vi "GraphsUpdateMai.vi"(0 "raw graph ref":refnum<vi>, 1 "File Paths":T3={"Local Save Path"=path "\\\\smbhome.uscs.susx.ac.uk\\cv222/Desktop/data", "Newton Save Path"=path "Z:/#Projects/Entanglement/data", "File Name"="test", "LocalSave"=TRUE}, 3 "Compiler Settings":T2={"Python Path"=path "", "Main File"="mainscript.py", "Meta File"="metascript.txt", "Aux File"="auxscript.py"}, 5 "mean graph ref":refnum<vi>, 7 "proc graph ref":refnum<vi>, 11 "error in (no error)":errorcluster, 12 "XControllerSettings":T1(xcontrol)) -> (15 "error out":errorcluster)   [LabVIEW 2017]
uses:
  controls/FilePaths.ctl
  PulseCompiler/CompilerSettings.ctl
  controls/xControllerSettings/XControllerSettings.xctl
  controls/GlobalExp.vi
  Global.lvlib
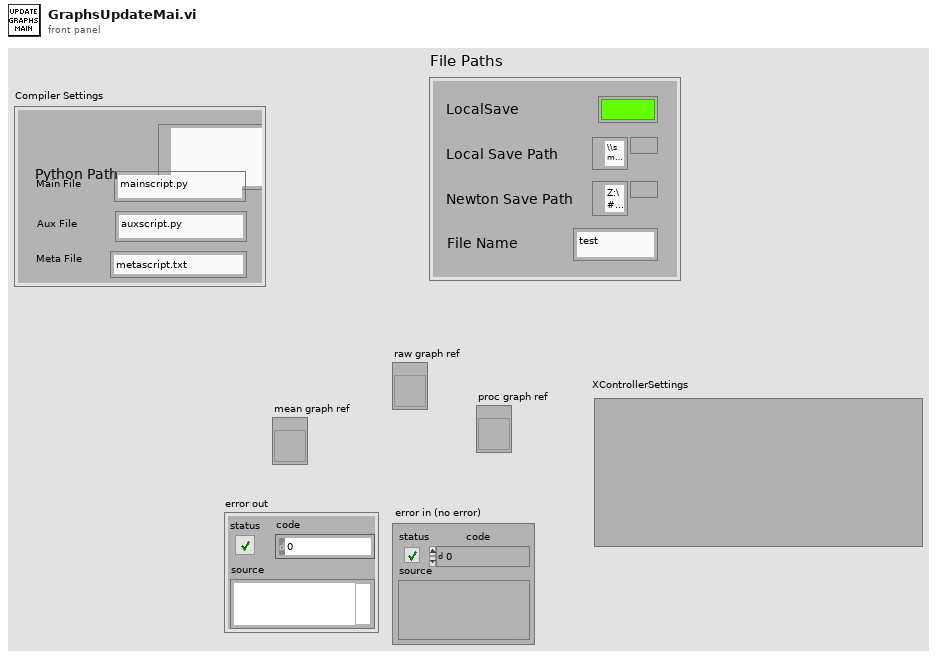
[diagram p1: front panel]
types:
  T1 = cluster{"Aux Sequence":bool, "Camera":bool, "Recrystallize":bool, "Raw graph":bool, "Mean graph":bool, "Calculate probs":bool, "Find fit":bool, "Dummy":bool}
  T2 = typedef "CompilerSettings.ctl" = cluster{"Python Path":path, "Main File":string, "Meta File":string, "Aux File":string}
  T3 = typedef "FilePaths.ctl" = cluster{"Local Save Path":path, "Newton Save Path":path, "File Name":string, "LocalSave":bool}
  T4 = typedef "MasterExpControl.ctl" = cluster{"Main Steps":dbl, "Main Runs":dbl, "ExpStatus":enum16{"Innit", "Stop", "Idle", "MainRunning", "AuxRunning"}, "Main Current Step":dbl, "ExpNum":dbl, "NewData":bool, "date":string, "command":string, "Stop":bool, "Pause":bool, "Mathematica":string, "Main/Meta":bool, "UpdateMath":bool, "Camera":bool, "MetaExpOver":bool}
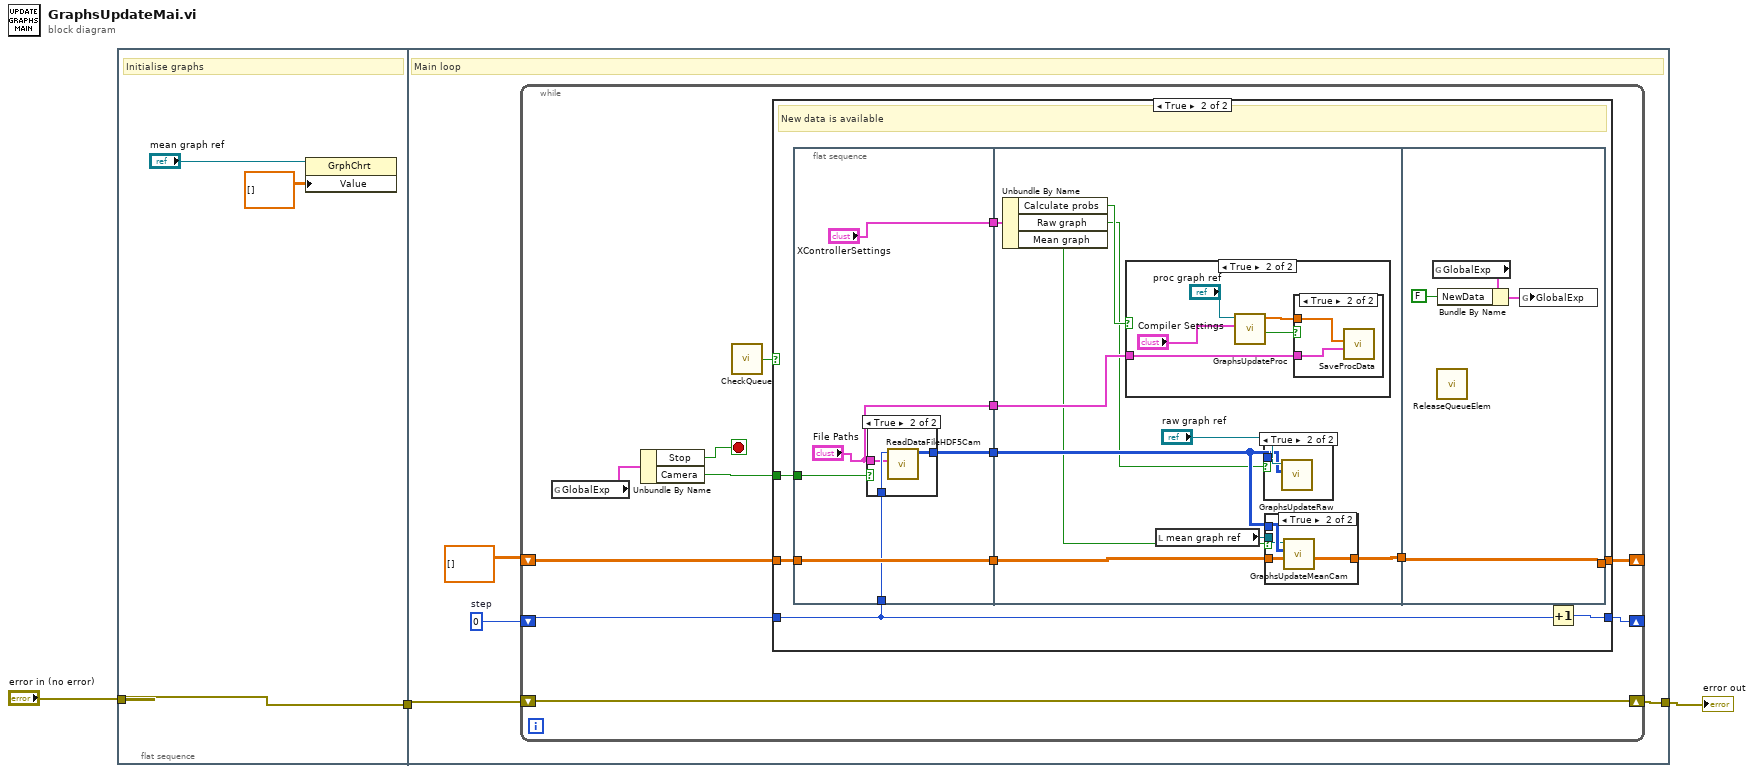
[diagram p0: block diagram]
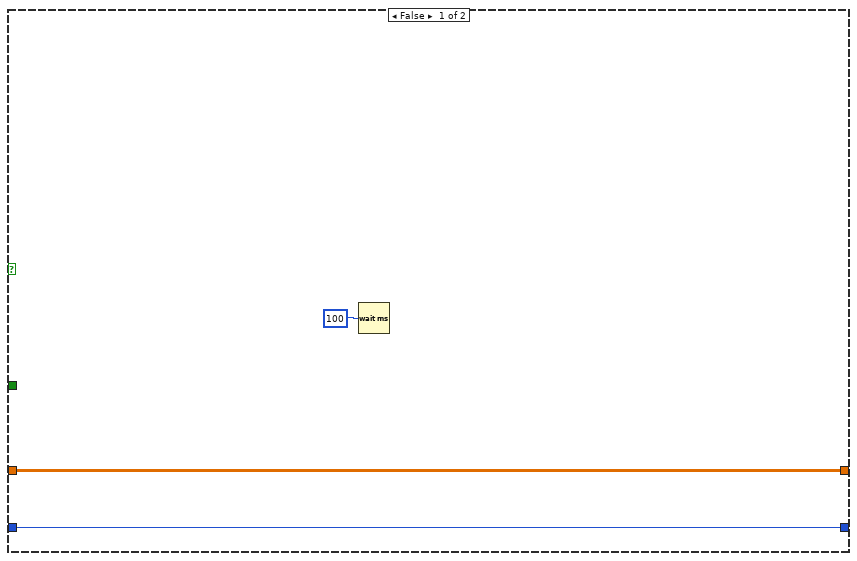
[diagram p2: hidden frame]
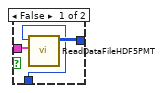
[diagram p3: hidden frame]
diagram:
  n1 = flat-sequence {
    tunnel: "error in (no error)" -> [w6]
    tunnel: [w6] -> w1
    tunnel: [w9] -> w2
    tunnel: w1 -> [w10]
    frame #0 {
      # "Initialise graphs"
      n2 = property class="GrphChrt"(reference="mean graph ref", "Value"=dbl[][] []) -> ()  [unwired: 1 in, 2 out]
    }
    frame #1 {
      w8 = 0  # step
      # "Main loop"
      n3 = while {
        shift-right: [w19] -> w9
        shift-left: w10 -> [w19]
        shift-right: [w13] -> _
        shift-left: w8 -> [w14]
        shift-right: [w11] -> _
        shift-left: dbl[][] [] -> [w12]
        stop <- w16 stop-if-true
        n4 = global read "GlobalExp.vi" "GlobalExp"() -> (w18:T4)
        n5 = Unbundle By Name(w18) -> ("Stop"=w16:bool, "Camera"=w17:bool)
        n6 = call "CheckQueue.vi"() -> ("x > 0?"=w15:bool)
        n7 = case shown="True" w15 {
          tunnel: w17 -> [_ w24]
          tunnel: w14 -> [w21 w29]
          tunnel: [w21 w32] -> w13
          tunnel: w12 -> [w20 w31]
          tunnel: [w20 w25] -> w11
          frame False {
            n8 = Wait (ms)(milliseconds to wait=u32 100) -> ()  [unwired: 1 out]
          }
          frame True {
            # "New data is available"
            n9 = flat-sequence {
              tunnel: w31 -> [w38]
              tunnel: [w38] -> w30
              tunnel: w29 -> [w37]
              tunnel: [w36] -> w28
              tunnel: ["File Paths"] -> w27
              tunnel: w24 -> [w34]
              tunnel: ["XControllerSettings"] -> w23
              tunnel: w30 -> [w54]
              tunnel: w28 -> [w51]
              tunnel: w27 -> [w52]
              tunnel: [w49] -> w26
              tunnel: w23 -> [w47]
              tunnel: w26 -> [w69]
              tunnel: [w69] -> w25
              frame #0 {
                n10 = case shown="True" w34 {
                  tunnel: w37 -> [w39 w44]
                  tunnel: [w41 w43] -> w36
                  tunnel: "File Paths" -> [w40 w42]
                  frame False {
                    n11 = call "ReadDataFileHDF5PMT.vi"("File Paths"=w40, "step"=w39) -> ("last step data"=w41:i32[][])  [unwired: 8 in, 1 out]
                  }
                  frame True {
                    n12 = call "ReadDataFileHDF5Cam.vi"("File Paths"=w42, "step"=w44) -> ("last step data"=w43:i32[][])  [unwired: 8 in, 1 out]
                  }
                }
              }
              frame #1 {
                n13 = Unbundle By Name(w47) -> ("Calculate probs"=w48:bool, "Raw graph"=w46:bool, "Mean graph"=w45:bool)
                n14 = case shown="True" w48 {
                  tunnel: w52 -> [_ w55]
                  frame False {
                  }
                  frame True {
                    n15 = call "GraphsUpdateProc.vi"("Compiler Settings"="Compiler Settings", "Prob graph ref in"="proc graph ref") -> ("SaveToCSV?"=w58:bool, "value"=w59:dbl[])  [unwired: 8 in]
                    n16 = case shown="True" w58 {
                      tunnel: w59 -> [_ w61]
                      tunnel: w55 -> [_ w60]
                      frame False {
                      }
                      frame True {
                        n17 = call "SaveProcData.vi"("File Paths"=w60, "probs list"=w61) -> ()  [unwired: 10 in]
                      }
                    }
                  }
                }
                n18 = local read "mean graph ref"() -> (w50:refnum<vi>)
                n19 = case shown="True" w46 {
                  tunnel: "raw graph ref" -> [_ w68]
                  tunnel: w51 -> [_ w67]
                  frame False {
                  }
                  frame True {
                    n20 = call "GraphsUpdateRaw.vi"("data in"=w67, "GraphChart in"=w68) -> ()  [unwired: 10 in]
                  }
                }
                n21 = case shown="True" w45 {
                  tunnel: w54 -> [w62 w66]
                  tunnel: w51 -> [_ w65]
                  tunnel: w50 -> [_ w64]
                  tunnel: [w62 w63] -> w49
                  frame False {
                  }
                  frame True {
                    n22 = call "GraphsUpdateMeanCam.vi"("Old mean data in"=w66, "run data in"=w65, "GraphChart in"=w64) -> ("New mean data out"=w63:dbl[][])  [unwired: 8 in]
                  }
                }
              }
              frame #2 {
                n23 = global read "GlobalExp.vi" "GlobalExp"() -> (w70:T4)
                n24 = call "ReleaseQueueElem.vi"() -> ()  [unwired: 12 in]
                n25 = Bundle By Name(cluster=w70, "NewData"=FALSE) -> (w71:T4)
                n26 = global write "GlobalExp.vi" "GlobalExp"(w71) -> ()
              }
            }
            n27 = Increment(x=w29) -> (x+1=w32:i32)
          }
        }
      }
    }
  }
  "error out" <- w2
